vi "Get DIO Lines from Ancestor.vi"(8 "error in":errorcluster, 11 "Bus Ref":refnum<data-value>) -> (0 "error out":errorcluster, 3 "DIO Lines":string[](array[string]))   [LabVIEW 2014, in "Device.lvclass"]
uses:
  Device.lvclass
  Bus/Bus.lvclass
  RIO Target/RIO Target.lvclass
  RIO Target Configuration/RIO Target Configuration.lvclass
  <vilib>/NI/Configuration Framework/Node/NISE_CEF_Node.lvclass/NISE_CEF_Node.ctl
  RIO Target Configuration/RIO Target Configuration.lvclass/RIO Target Configuration.ctl
  <vilib>/NI/Configuration Framework/Node/ReadParent.vi
  <vilib>/NI/Configuration Framework/Node/NISE_CEF_Node.lvclass
  <vilib>/NI/Configuration Framework/serializable configuration/NISE_CEF_serializable configuration.lvclass
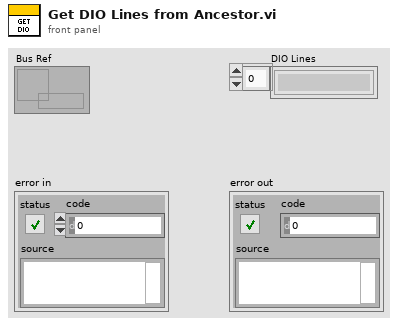
[diagram p1: front panel]
types:
  T1 = typedef "NISE_CEF_Node.lvclass/NodeRef.ctl" = refnum<data-value>
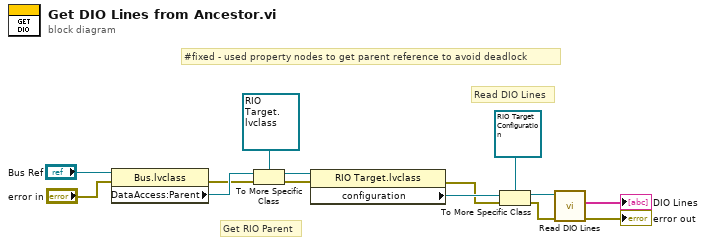
[diagram p0: block diagram]
diagram:
  # "#fixed - used property nodes to get parent reference to avoid deadlock"
  # "Read DIO Lines"
  # "Get RIO Parent"
  n1 = property class="Bus.lvclass"(reference="Bus Ref", error in="error in") -> (error out=w10:errorcluster, "DataAccess:Parent"=w11:T1)  [unwired: 1 out]
  n2 = To More Specific Class(target class=refnum<data-value> refnum ("data value reference"), reference=w11, error in=w10) -> (specific class reference=w9:refnum<data-value>, error out=w5:errorcluster)
  n3 = property class="RIO Target.lvclass"(reference=w9, error in=w5) -> (error out=w3:errorcluster, "configuration"=w4:refnum<class "NISE_CEF_serializable configuration.lvclass">)  [unwired: 1 out]
  n4 = To More Specific Class(target class=refnum<class "RIO Target Configuration.lvclass"> refnum ("RIO Target Configuration in"), reference=w4, error in=w3) -> (specific class reference=w7:refnum<class "RIO Target Configuration.lvclass">, error out=w6:errorcluster)
  n5 = call "Read DIO Lines.vi"("error in (no error)"=w6, "RIO Target Configuration in"=w7) -> ("error out"=→"error out":errorcluster, "DIO Lines"=→"DIO Lines":string[])  [unwired: 7 in, 1 out]
